vi "Build Exp Wvfrm (Wvfrm).vi"(8 "error in (no error)":errorcluster, 9 "Express Waveform Attributes":T1 {"Timestamp" format="%<%X\n%x>T"; "Start Timestamp" format="%<%X\n%x>T"}, 11 "Waveform":waveform(dbl)) -> (0 "error out":errorcluster, 3 "Waveform":waveform(dbl))   [LabVIEW 2020]
uses:
  <vilib>/express/express shared/transition.llb/ex_WaveformAttribs.ctl
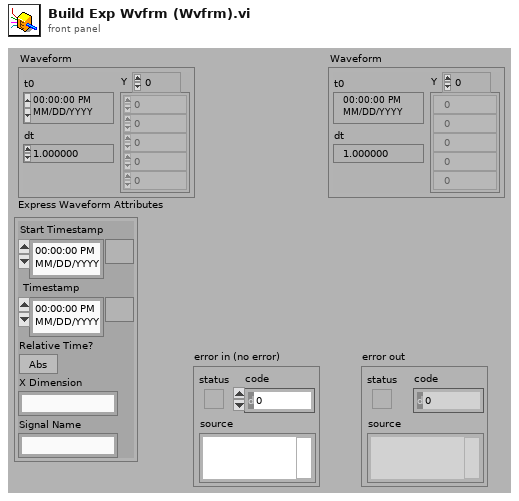
[diagram p1: front panel]
types:
  T1 = typedef "ex_WaveformAttribs.ctl" = cluster{"Start Timestamp":timestamp, "Timestamp":timestamp, "Relative Time?":bool, "X Dimension":string, "Signal Name":string}
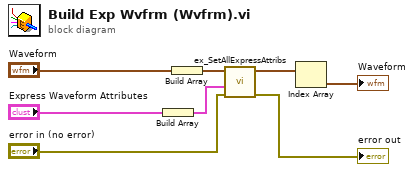
[diagram p0: block diagram]
diagram:
  n1 = Build Array("Express Waveform Attributes") -> (w7:T1[])
  n2 = Build Array("Waveform") -> (w6:waveform(dbl)[])
  n3 = call <vilib>:"ex_SetAllExpressAttribs.vi"("error in"="error in (no error)", "All Express Wave Attributes"=w7, "Signals"=w6) -> ("error out"=→"error out":errorcluster, "Signals With Attributes"=w5:waveform(dbl)[])  [unwired: 7 in]
  n4 = Index Array(array=w5) -> (element=→"Waveform":waveform(dbl))  [unwired: 1 in]
